vi "FTW-ERR-ThrowWarning.vi"(7 "Warning Message":string, 9 "Error Code":i32, 11 "error in":errorcluster) -> (15 "error out":errorcluster)   [LabVIEW 2015]
doc: "Throws an error if the \"Error Code\" input is non-zero."
panel:
  # "Inputs"
  # "Outputs"
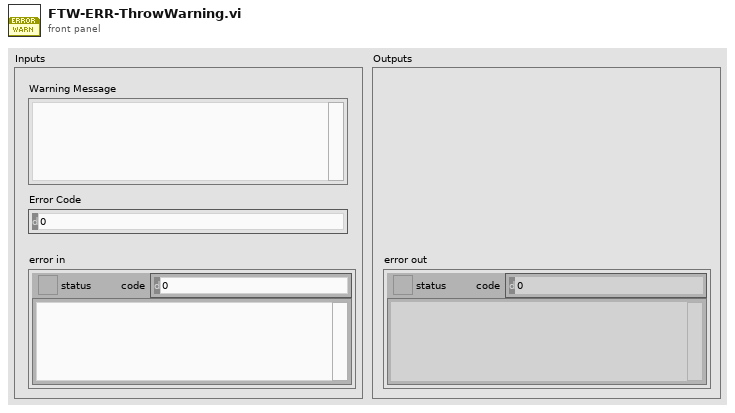
[diagram p1: front panel]
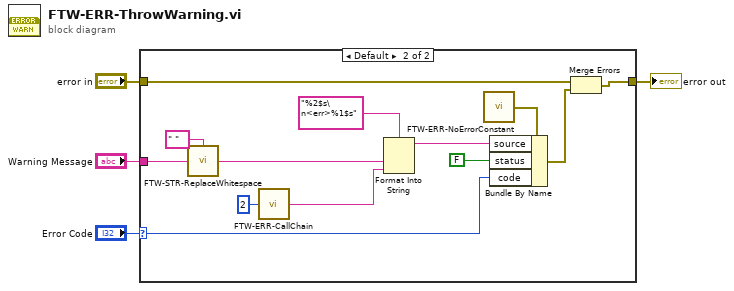
[diagram p0: block diagram]
diagram:
  n1 = case shown="Default" "Error Code" {
    selector: "Error Code" -> [_ w9]
    tunnel: "error in" -> [w5 w17]
    tunnel: [w5 w16] -> w3
    tunnel: "Warning Message" -> [_ w8]
    frame 0 {
    }
    frame Default {
      n2 = call "FTW-STR-ReplaceWhitespace.vi"("Replace Spaces With..."=" " ("String"), "Input"=w8) -> ("Output"=w7:string)  [unwired: 2 in]
      n3 = call "FTW-ERR-CallChain.vi"("Levels to exclude (1=This VI's caller)"=2) -> ("Call Chain"=w10:string)
      n4 = Format Into String(format string="%2$s\n<err>%1$s", w7, w10) -> (resulting string=w12:string)  [unwired: 2 in, 1 out]
      n5 = call "FTW-ERR-NoErrorConstant.vi"() -> ("no error"=w11:errorcluster)
      n6 = Bundle By Name(cluster=w11, "source"=w12, "status"=FALSE, "code"=w9) -> (w18:errorcluster)
      n7 = Merge Errors(w17, w18) -> (w16:errorcluster)
    }
  }
  "error out" <- w3
